vi "Template Response (Path).vi"(8 "error in (no error)":errorcluster, 10 "Template Path":path, 11 "Processing in":refnum<class "Processing.lvclass">) -> (0 "error out":errorcluster, 3 "Processing out":refnum<class "Processing.lvclass">)   [LabVIEW 2020, in "HTTP Server.lvlib" / "Processing.lvclass"]
uses:
  Processing.lvclass
  Processing.lvclass/Processing.ctl
  lv-http-util/HTTP Utils/Response/Response.lvclass
panel:
  in  "Content-Type (text/html)":string="text/html"
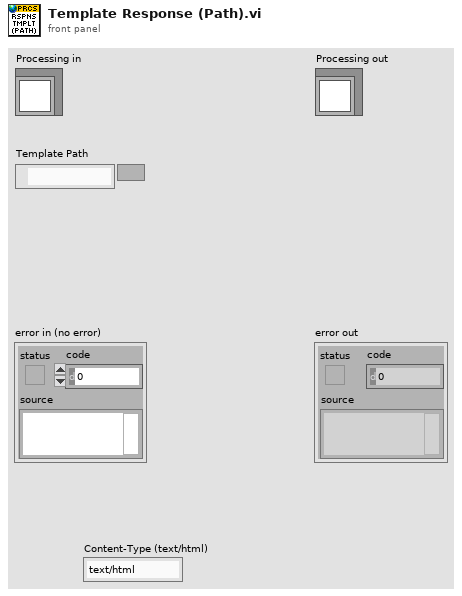
[diagram p1: front panel]
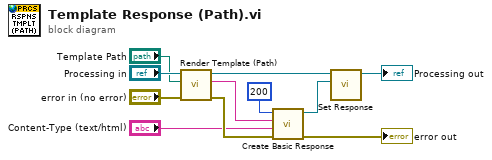
[diagram p0: block diagram]
diagram:
  n1 = call "Render Template (Path).vi"("error in (no error)"="error in (no error)", "Path"="Template Path", "Processing in"="Processing in") -> ("error out"=w11:errorcluster, "String"=w1:string, "Processing out"=w2:refnum<class "Processing.lvclass">)  [unwired: 6 in]
  n2 = call "Create Basic Response.vi"("error in (no error)"=w11, "Content-Type (text/plain)"="Content-Type (text/html)", "Payload"=w1, "Status Code"=u16 200) -> ("error out"=→"error out":errorcluster, "Response out"=w8:refnum<class "Response.lvclass">)  [unwired: 6 in]
  n3 = call "Set Response.vi"("Response"=w8, "Processing in"=w2) -> ("Processing out"=→"Processing out":refnum<class "Processing.lvclass">)  [unwired: 9 in]
